vi "orbit fitter.vi"(8 "error in (no error)":errorcluster, 10 "crossing stats":T4, 11 "display queues":T2) -> (0 "error out":errorcluster, 3 "elliptical fit":T1)   [LabVIEW 2017]
uses:
  typedefs/queue cluster.ctl
  typedefs/reading queue.ctl
  typedefs/reading.ctl
  typedefs/readingType.ctl
  typedefs/magnetomter reading set.ctl
  typedefs/magnet location with timestamp.ctl
  typedefs/orbit parameters full.ctl
panel:
  in  "initialize with prev fit results":bool
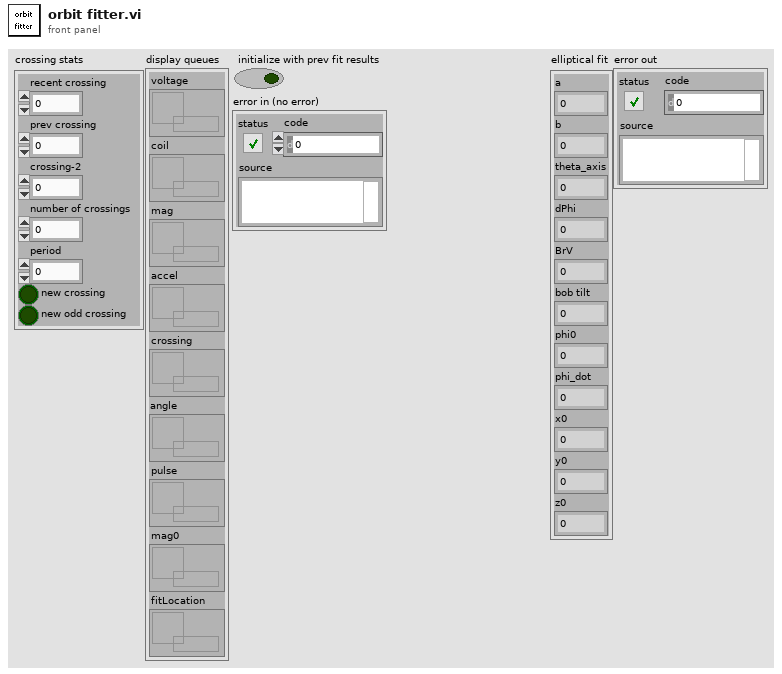
[diagram p1: front panel]
types:
  T1 = typedef "orbit parameters full.ctl" = cluster{"a":dbl, "b":dbl, "theta_axis":dbl, "dPhi":dbl, "BrV":dbl, "bob tilt":dbl, "phi0":dbl, "phi_dot":dbl, "x0":dbl, "y0":dbl, "z0":dbl}
  T2 = typedef "queue cluster.ctl" = cluster{"voltage":T3, "coil":T3, "mag":refnum<queue>, "accel":T3, "crossing":T3, "angle":T3, "pulse":T3, "mag0":T3, "fitLocation":refnum<queue>}
  T3 = typedef "reading queue.ctl" = refnum<queue>
  T4 = cluster{"recent crossing":dbl, "prev crossing":dbl, "crossing-2":dbl, "number of crossings":i32, "period":dbl, "new crossing":bool, "new odd crossing":bool}
  T5 = typedef "magnetomter reading set.ctl" = cluster{"time":fxp<+,48,48>, "mag readings":cluster{"magnetometer index":dbl, "Bx":dbl, "By":dbl, "Bz":dbl, "magnetometer x":dbl, "magnetometer y":dbl}[]}
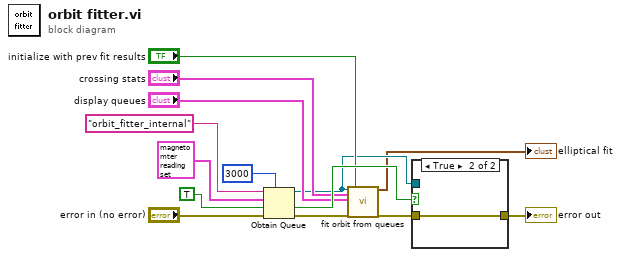
[diagram p0: block diagram]
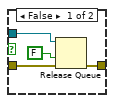
[diagram p2: hidden frame]
diagram:
  n1 = Obtain Queue(max queue size (-1, unlimited)=3000, name (unnamed)="orbit_fitter_internal", element data type=T5 {"time"=0.0, "mag readings"=[]} ("Magnetometer reading set"), create if not found? (T)=TRUE, error in (no error)="error in (no error)") -> (queue out=w4:refnum<queue>, created new?=w10:bool, error out=w6:errorcluster)
  n2 = call "fit orbit from queues.vi"("magnetometer set queue"=w4, "crossing stats"="crossing stats", "display queues"="display queues", "error in (no error)"=w6, "initialize with prev fit results"="initialize with prev fit results") -> ("elliptical fit"=→"elliptical fit":T1, "error out"=w5:errorcluster)  [unwired: 13 in]
  n3 = case shown="True" w10 {
    tunnel: w5 -> [w16 w19]
    tunnel: w4 -> [w18 _]
    tunnel: [w15 w19] -> w1
    frame False {
      n4 = Release Queue(queue=w18, force destroy? (F)=FALSE, error in (no error)=w16) -> (error out=w15:errorcluster)  [unwired: 2 out]
    }
    frame True {
    }
  }
  "error out" <- w1
